vi "Mixer Example.vi"() -> ()   [LabVIEW 2020]
uses:
  Mixer/Channel/Controls/Channel State.ctl
  Mixer/Mixer/Polymorphic VIs/Channel Load (Path).vi
  Mixer/Mixer/Mixer.lvclass
  Mixer/Channel/Channel.lvclass
panel:
  out "State 3":T1
  out "State 2":T1
  out "State 1":T1
  out "State 0":T1
  in  "Pause -1":bool
  in  "Stop -1":bool
  in  "Exit":bool
  in  "Path 3":path
  in  "Path 2":path
  in  "Path 1":path
  in  "Path 0":path
  in  "Play -1":bool
  in  "Volume 3":sgl(slide)=1.0 scale=0.0..2.0
  in  "Volume 2":sgl(slide)=1.0 scale=0.0..2.0
  in  "Volume 1":sgl(slide)=1.0 scale=0.0..2.0
  in  "Volume 0":sgl(slide)=1.0 scale=0.0..2.0
  in  "Pause 3":bool
  in  "Pause 2":bool
  in  "Pause 1":bool
  in  "Pause 0":bool
  in  "Stop 3":bool
  in  "Stop 2":bool
  in  "Stop 1":bool
  in  "Stop 0":bool
  in  "Play 3":bool
  in  "Play 2":bool
  in  "Play 1":bool
  in  "Play 0":bool
  # "Instructions:\n1. Run the VI.\n2. Select an audio file to play.\n3. The VI will stop when the file has finished playing, or when the Stop button is pressed."
  # "Tip: Press keys 1-4 to play the corresponding channel. Pressing the key or the Play button during playback will retrigger the sample."
  # "G"
  # "-Audio"
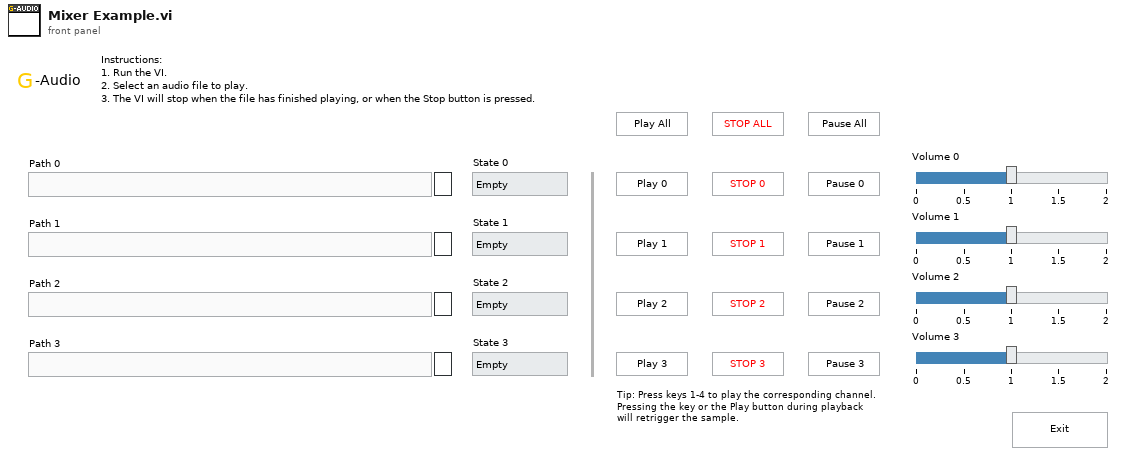
[diagram p1: front panel]
types:
  T1 = typedef "G-Audio.lvlib/Channel.lvclass/Channel State.ctl" = enum16{"Empty", "Error", "Loading", "Loaded", "Stopped", "Paused", "Playing", "Retrigger"}
  T2 = typedef "G-Audio.lvlib/Channel.lvclass/Channel Status.ctl" = cluster{"Frame":u64, "State":T1, "Volume":dbl}
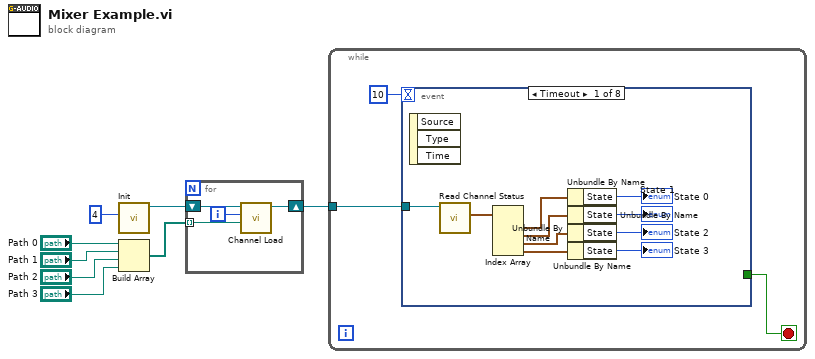
[diagram p0: block diagram]
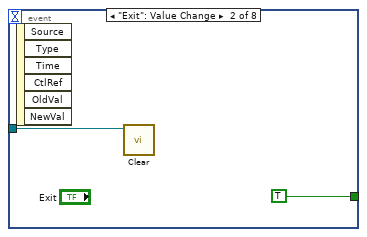
[diagram p2: hidden frame]
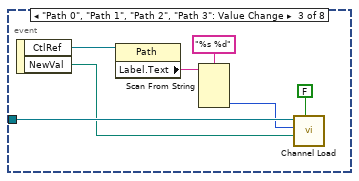
[diagram p3: hidden frame]
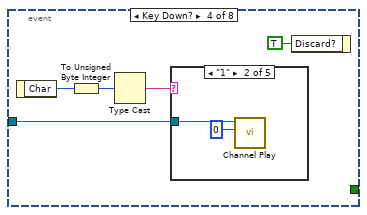
[diagram p4: hidden frame]
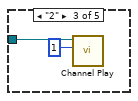
[diagram p6: hidden frame]
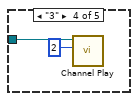
[diagram p7: hidden frame]
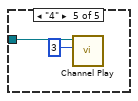
[diagram p8: hidden frame]
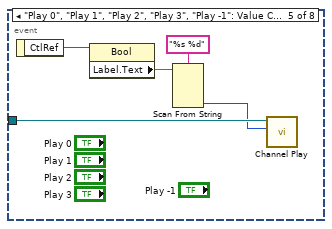
[diagram p9: hidden frame]
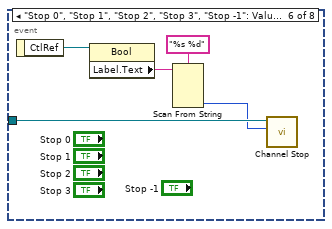
[diagram p10: hidden frame]
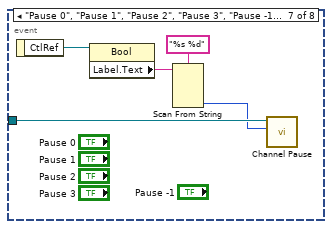
[diagram p11: hidden frame]
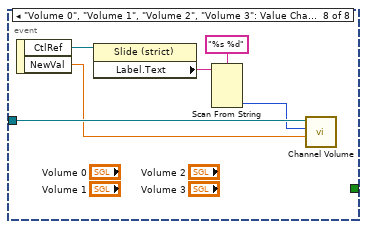
[diagram p12: hidden frame]
diagram:
  n1 = call "Init.vi"("Channel Count (16)"=4) -> ("Mixer out"=w8:refnum<class "Mixer.lvclass">)  [unwired: 9 in, 1 out]
  n2 = Build Array("Path 0", "Path 1", "Path 2", "Path 3") -> (w3:path[])
  n3 = for {
    shift-right: [w11] -> w2
    shift-left: w8 -> [w12]
    tunnel: w3 -> [w10] mode=indexing
    i -> [w9]
    n4 = call-poly "Channel Load.vi"("Path"=w10, "Channel Index"=w9, "Mixer in"=w12) -> ("Mixer out"=w11:refnum<class "Mixer.lvclass">)  [unwired: 7 in, 1 out]
  }
  n5 = while {
    tunnel: w2 -> [w15]
    stop <- w14 stop-if-true
    n6 = event shown="[0] Timeout" {
      selector: _ -> [_ _ _ _ _ _ _ _]
      dyn-events: _ -> [_ _ _ _ _ _ _ _]
      timeout: 10 -> [_ _ _ _ _ _ _ _]
      tunnel: w15 -> [w25 w27 w34 w37 w52 w57 w62 w68]
      tunnel: [_ TRUE _ _ _ _ _ _] -> w14
      event Timeout {
        n7 = event-data() -> ()  [unwired: 1 in, 3 out]
        n8 = call "Read Channel Status.vi"("Mixer in"=w25) -> ("Channel Status"=w24:T2[])  [unwired: 8 in, 2 out]
        n9 = Index Array(array=w24) -> (element #1=w23:T2, element #2=w20:T2, element #3=w21:T2, element #4=w22:T2)  [unwired: 4 in]
        n10 = Unbundle By Name(w23) -> ("State"=→"State 0":T1)
        n11 = Unbundle By Name(w20) -> ("State"=→"State 1":T1)
        n12 = Unbundle By Name(w21) -> ("State"=→"State 2":T1)
        n13 = Unbundle By Name(w22) -> ("State"=→"State 3":T1)
      }
      event "Exit": Value Change {
        n14 = event-data() -> ()  [unwired: 1 in, 6 out]
        n15 = call "Clear.vi"("Mixer in"=w27) -> ()  [unwired: 10 in, 1 out]
      }
      event "Path 0", "Path 1", "Path 2", "Path 3": Value Change {
        n16 = event-data() -> ("CtlRef"=w31:refnum<vi>, "NewVal"=w30:path)  [unwired: 1 in]
        n17 = property class="Path"(reference=w31) -> ("Label.Text"=w33:string)  [unwired: 1 in, 2 out]
        n18 = Scan From String(format string="%s %d", input string=w33) -> (output 2=w28:i32)  [unwired: 5 in, 3 out]
        n19 = call-poly "Channel Load.vi"("Wait For Load (T)"=FALSE, "Path"=w30, "Channel Index"=w28, "Mixer in"=w34) -> ()  [unwired: 6 in, 2 out]
      }
      event Key Down? {
        n20 = event-data() -> ("Char"=w38:i16)  [unwired: 1 in]
        n21 = To Unsigned Byte Integer(number=w38) -> (unsigned 8bit integer=w36:u8)
        n22 = Type Cast(x=w36) -> (*(type *) &x=w35:string)  [unwired: 1 in]
        n23 = case shown="\"1\"" w35 {
          tunnel: w37 -> [_ w41 w43 w45 w47]
          frame Default {
          }
          frame "1" {
            n24 = call "Channel Play.vi"("Channel Index"=0, "Mixer in"=w41) -> ()  [unwired: 8 in, 2 out]
          }
          frame "2" {
            n25 = call "Channel Play.vi"("Channel Index"=1, "Mixer in"=w43) -> ()  [unwired: 8 in, 2 out]
          }
          frame "3" {
            n26 = call "Channel Play.vi"("Channel Index"=2, "Mixer in"=w45) -> ()  [unwired: 8 in, 2 out]
          }
          frame "4" {
            n27 = call "Channel Play.vi"("Channel Index"=3, "Mixer in"=w47) -> ()  [unwired: 8 in, 2 out]
          }
        }
        n28 = event-data("Discard?"=TRUE) -> ()  [unwired: 1 in, 1 out]
      }
      event "Play 0", "Play 1", "Play 2", "Play 3", "Play -1": Value Change {
        n29 = event-data() -> ("CtlRef"=w51:refnum<vi>)  [unwired: 1 in]
        n30 = property class="Bool"(reference=w51) -> ("Label.Text"=w50:string)  [unwired: 1 in, 2 out]
        n31 = Scan From String(format string="%s %d", input string=w50) -> (output 2=w48:i32)  [unwired: 5 in, 3 out]
        n32 = call "Channel Play.vi"("Channel Index"=w48, "Mixer in"=w52) -> ()  [unwired: 8 in, 2 out]
      }
      event "Stop 0", "Stop 1", "Stop 2", "Stop 3", "Stop -1": Value Change {
        n33 = event-data() -> ("CtlRef"=w56:refnum<vi>)  [unwired: 1 in]
        n34 = property class="Bool"(reference=w56) -> ("Label.Text"=w55:string)  [unwired: 1 in, 2 out]
        n35 = Scan From String(format string="%s %d", input string=w55) -> (output 2=w53:i32)  [unwired: 5 in, 3 out]
        n36 = call "Channel Stop.vi"("Channel Index"=w53, "Mixer in"=w57) -> ()  [unwired: 8 in, 2 out]
      }
      event "Pause 0", "Pause 1", "Pause 2", "Pause 3", "Pause -1": Value Change {
        n37 = event-data() -> ("CtlRef"=w61:refnum<vi>)  [unwired: 1 in]
        n38 = property class="Bool"(reference=w61) -> ("Label.Text"=w60:string)  [unwired: 1 in, 2 out]
        n39 = Scan From String(format string="%s %d", input string=w60) -> (output 2=w58:i32)  [unwired: 5 in, 3 out]
        n40 = call "Channel Pause.vi"("Channel Index"=w58, "Mixer in"=w62) -> ()  [unwired: 8 in, 2 out]
      }
      event "Volume 0", "Volume 1", "Volume 2", "Volume 3": Value Change {
        n41 = event-data() -> ("CtlRef"=w67:refnum<vi>, "NewVal"=w64:sgl)  [unwired: 1 in]
        n42 = property class="Slide (strict)"(reference=w67) -> ("Label.Text"=w66:string)  [unwired: 1 in, 2 out]
        n43 = Scan From String(format string="%s %d", input string=w66) -> (output 2=w63:i32)  [unwired: 5 in, 3 out]
        n44 = call "Channel Volume.vi"("Volume"=w64, "Channel Index"=w63, "Mixer in"=w68) -> ()  [unwired: 7 in, 2 out]
      }
    }
  }
